vi "LVClass_HasoField Get Max Size.vi"(0 "HasoField in":refnum<class "HasoField.lvclass">, 11 "error in (no error)":errorcluster) -> (4 "HasoField out":refnum<class "HasoField.lvclass">, 8 "MaxSize":u32, 15 "error out":errorcluster)   [LabVIEW 2020, in "HasoField.lvclass"]
doc: "Get the wavelength of the source.\n\n--------------------------------------------------------------------------------\n\n<B>HasoFieldIn </B> : HasoField object.\n<B>HasoFieldOut </B> : HasoField object.\n<B>wavelength </B> : Wavelength of the source.\n<B>ErrorIn </B> : Error\n<B>ErrorOut </B> : Error\n\n--------------------------------------------------------------------------------"
uses:
  HasoField.lvclass
  HasoField.lvclass/HasoField.ctl
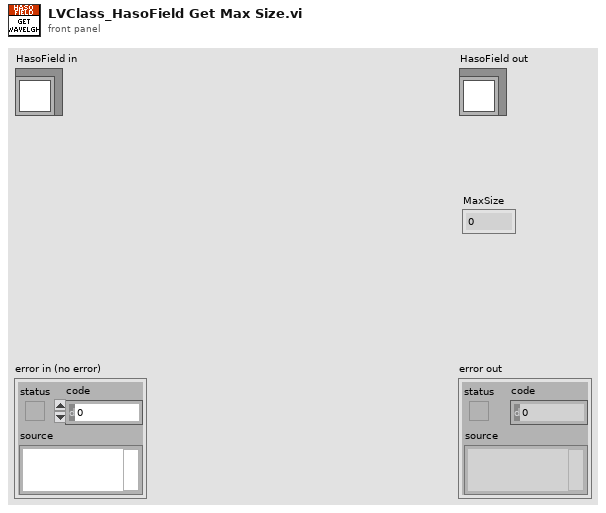
[diagram p1: front panel]
types:
  T1 = typedef "ClassID.ctl" = i64
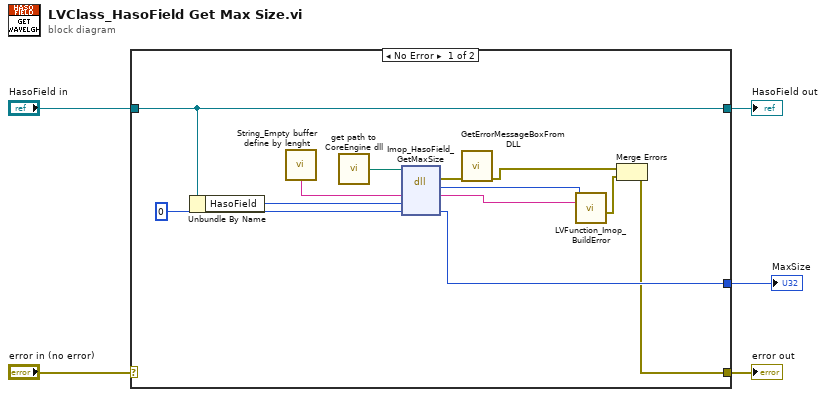
[diagram p0: block diagram]
diagram:
  n1 = case shown="No Error" "error in (no error)" {
    selector: "error in (no error)" -> [_ w19]
    tunnel: [w6 w19] -> w4
    tunnel: [w9 w18] -> w2
    tunnel: "HasoField in" -> [w9 w18]
    tunnel: [w7 _] -> w1
    frame No Error {
      n2 = Unbundle By Name(w9) -> ("HasoField"=w8:T1)
      n3 = call "String_Empty buffer define by lenght.vi"() -> ("Empty buffer"=w13:string)  [unwired: 1 in]
      n4 = call "get path to CoreEngine dll.vi"() -> ("path to wavekit library"=w12:path)  [unwired: 14 in, 1 out]
      n5 = dll-call lib="D:/soft/HASO_v3/SVN_trunk/ImOpCoreEngine4_LV2011/DLLs/c_interface_vc100.dll" fn="Imop_HasoField_GetMaxSize"(path in=w12, "message"=w13, "HasoField"=w8, "MaxSize"=u32 0 ("wavelength")) -> (error out=w11:errorcluster, "return type"=w16:i32, "message"=w17:string, "MaxSize"=w7:u32)  [unwired: 3 in, 1 out]
      n6 = call "GetErrorMessageBoxFromDLL.vi"("error IN"=w11) -> ("error OUT"=w15:errorcluster)  [unwired: 10 in]
      n7 = call "LVFunction_Imop_BuildError.vi"("code"=w16, "String to Prepend to source (\"\")"=w17) -> ("error out"=w14:errorcluster)  [unwired: 13 in]
      n8 = Merge Errors(w15, w14) -> (w6:errorcluster)
    }
    frame Error {
    }
  }
  "error out" <- w4
  "HasoField out" <- w2
  "MaxSize" <- w1
